vi "clearpath_parse_safety_status.vi"(0 "ClearpathComm":T1) -> (1 "Data Valid?":bool=TRUE, 2 "Flags":u8 format="%x")   [LabVIEW 2012, in "clearpath_interface.lvlib"]
doc: "Parses current status of platform safety system. (Message type 0x8010)"
uses:
  IGVC/Clearpath/Husky 2011/Teleop Robotics Project Folder/Husky/vi/clearpath_interface.lvlib
  cwrap_crio.dll
panel:
  # "Safety System Status"
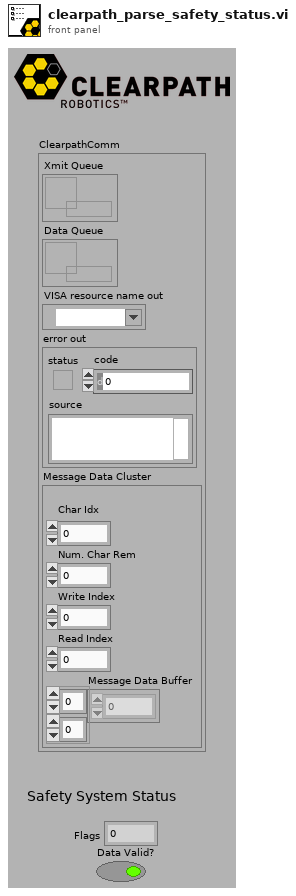
[diagram p1: front panel]
types:
  T1 = cluster{"Xmit Queue":refnum<queue>, "Data Queue":refnum<queue>, "VISA resource name out":refnum<visa-resource-name>, "error out":errorcluster, "Message Data Cluster":cluster{"\nChar Idx":u8, "Num. Char Rem":u8, "Write Index":u8, "Read Index":u8, "Message Data Buffer":u8[][]}}
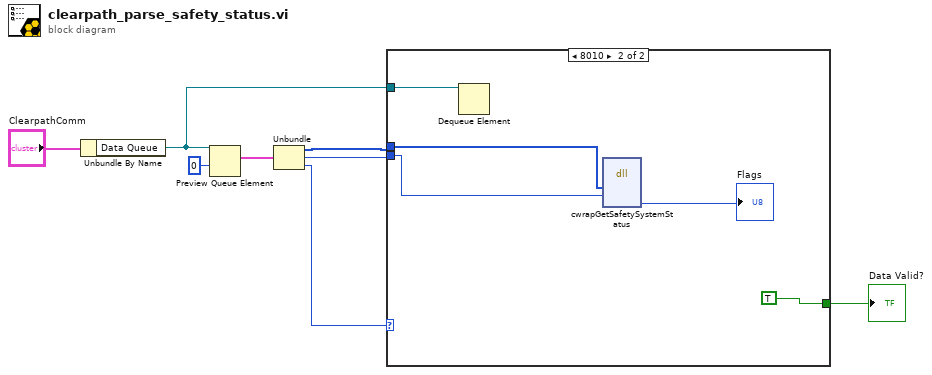
[diagram p0: block diagram]
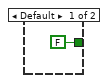
[diagram p2: hidden frame]
diagram:
  n1 = Unbundle By Name("ClearpathComm") -> ("Data Queue"=w1:refnum<queue>)
  n2 = Preview Queue Element(queue=w1, timeout in ms (-1)=0) -> (element=w6:cluster{u8[], "Length":i32, "Type":i32})  [unwired: 1 in, 3 out]
  n3 = Unbundle(w6) -> (w3:u8[], "Length"=w4:i32, "Type"=w5:i32)
  n4 = case shown="8010" w5 {
    tunnel: w4 -> [_ w12]
    tunnel: w3 -> [_ w13]
    tunnel: [FALSE TRUE] -> w2
    tunnel: w1 -> [_ w10]
    frame Default {
    }
    frame 32784 {
      n5 = Dequeue Element(queue=w10) -> ()  [unwired: 2 in, 4 out]
      n6 = dll-call lib="C:/Users/tebbeam/Documents/GitHub/IGVC-2013/Code/Project 1.0/Motors/Husky/cwrap_cRIO.*" fn="cwrapGetSafetySystemStatus"("packet"=w13, "len"=w12) -> ("flags"=→"Flags":u8)  [unwired: 7 in, 2 out]
    }
  }
  "Data Valid?" <- w2
